vi "Get Device USB Strings.vi"(8 "error in (no error)":errorcluster, 11 "Device Index":u32) -> (0 "error out":errorcluster, 2 "function return":i32, 3 "Device USB Strings":T1)   [LabVIEW 2016]
doc: "Retrieves manufacturer, product, and serial number from the device specified by index."
uses:
  Controls/Device USB String.ctl
panel:
  in  "serial":string
  in  "product":string
  in  "manufact":string
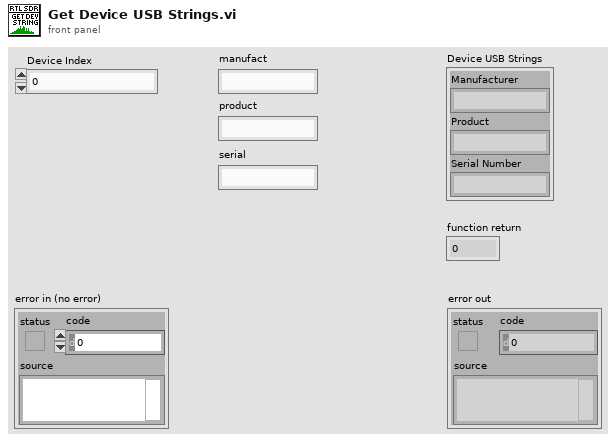
[diagram p1: front panel]
types:
  T1 = typedef "Device USB String.ctl" = cluster{"Manufacturer":string, "Product":string, "Serial Number":string}
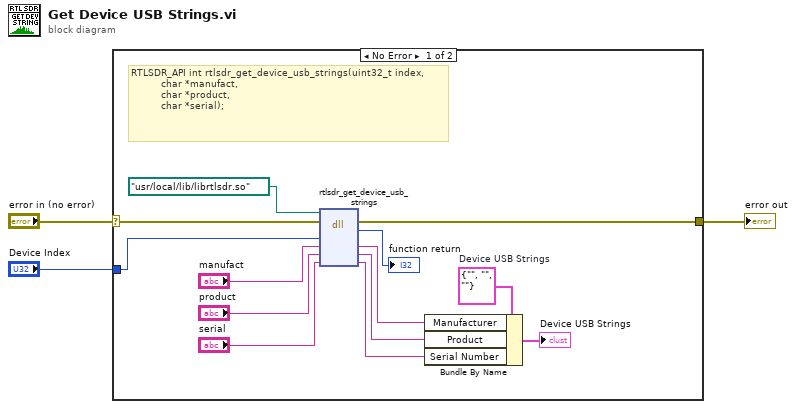
[diagram p0: block diagram]
diagram:
  n1 = case shown="No Error" "error in (no error)" {
    selector: "error in (no error)" -> [w7 w17]
    tunnel: "Device Index" -> [w6 _]
    tunnel: [w12 w17] -> w2
    frame No Error {
      w5 = T1 {"Manufacturer"="", "Product"="", "Serial Number"=""}  # Device USB Strings
      # "RTLSDR_API int rtlsdr_get_device_usb_strings(uint32_t index,\n\t\t\t\t\t     char *manufact,\n\t\t\t\t\t     char *product,\n\t\t\t\t\t     char *serial);"
      n2 = dll-call lib="C:/Program Files (x86)/National Instruments/LabVIEW 2016/user.lib/rtlsdr/rtlsdr.*" fn="rtlsdr_get_device_usb_strings"(path in=path "/usr/local/lib/librtlsdr.so", error in=w7, "index"=w6, "manufact"="manufact", "product"="product", "serial"="serial") -> (error out=w12:errorcluster, "return type"=→"function return":i32, "manufact"=w10:string, "product"=w9:string, "serial"=w8:string)  [unwired: 2 in, 1 out]
      n3 = Bundle By Name(cluster=w5, "Manufacturer"=w10, "Product"=w9, "Serial Number"=w8) -> (→"Device USB Strings":T1)
    }
    frame Error {
    }
  }
  "error out" <- w2
